vi "Next.vi"(8 "error in (no error)":errorcluster, 11 "Runnable In":refnum<class "Runnable.lvclass">) -> (0 "error out":errorcluster, 1 "Suite":string, 2 "Name":string, 3 "Runnable Out":refnum<class "Runnable.lvclass">)   [LabVIEW 2020, in "Runnable.lvclass"]
uses:
  Runnable.lvclass
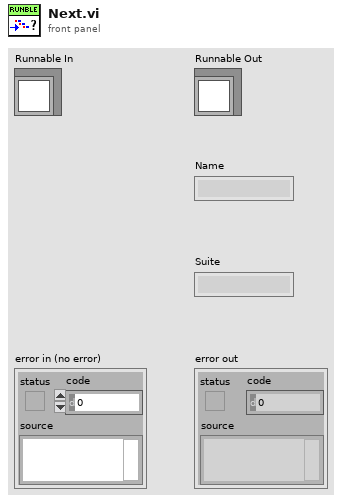
[diagram p1: front panel]
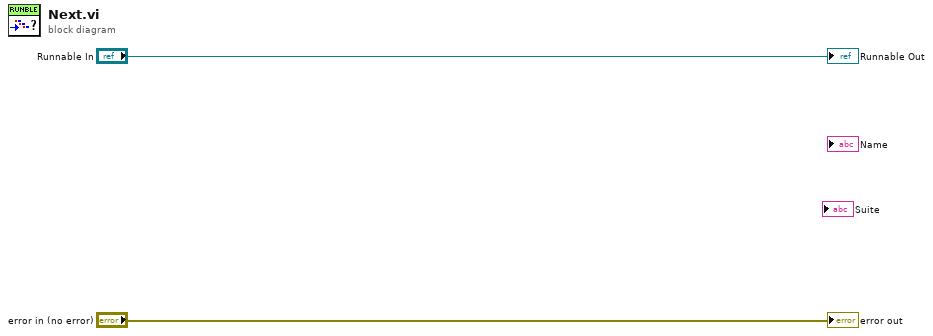
[diagram p0: block diagram]
diagram:
  "error out" <- "error in (no error)"
  "Runnable Out" <- "Runnable In"
